vi "Global 1.vi"() -> ()   [LabVIEW 2022 SP3]
panel:
  in  "Numeric":i32=10
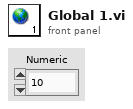
[diagram p1: front panel]
diagram:
